vi "GDFgetEventTable.vi"(8 "error in (no error)":errorcluster, 11 "GDFv1.x in":refnum<class "GDFv1.x.lvclass">) -> (0 "error out":errorcluster, 2 "Event Table":T1[](array[typedef]), 3 "GDFv1.x out":refnum<class "GDFv1.x.lvclass">)   [LabVIEW 2016, in "GDF File Reader.lvlib" / "GDFv1.x.lvclass"]
uses:
  GDFv1.x.lvclass
  EventDataType.ctl
  GDFv1.x.lvclass/GDFv1.x.ctl
  GDF File Reader.lvlib
panel:
  # "This VI is a part of BCI Design library, http://www.ru-bci.org \nCopyright © 2020, Sotnikov Peter, All rights reserved. License: GNU GPLv3"
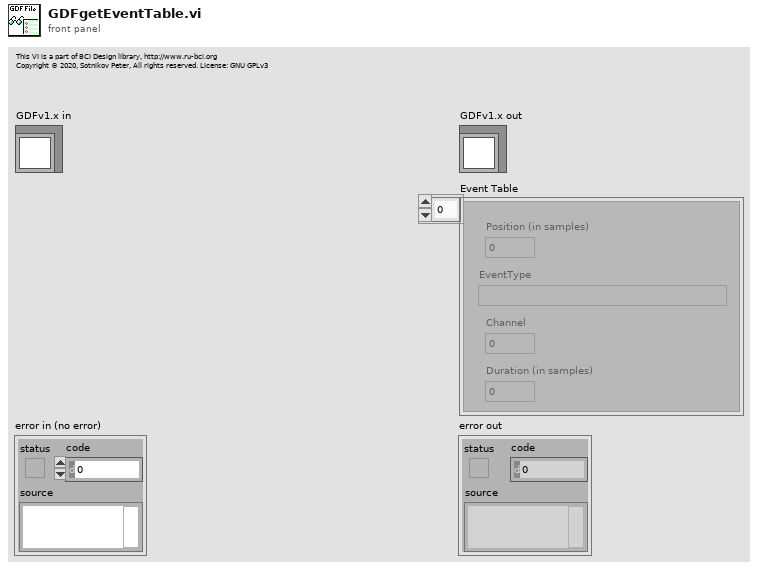
[diagram p1: front panel]
types:
  T1 = typedef "GDF File Reader.lvlib/EventDataType.ctl" = cluster{"Position (in samples)":u32, "EventType":string, "Channel":u16, "Duration (in samples)":u32}
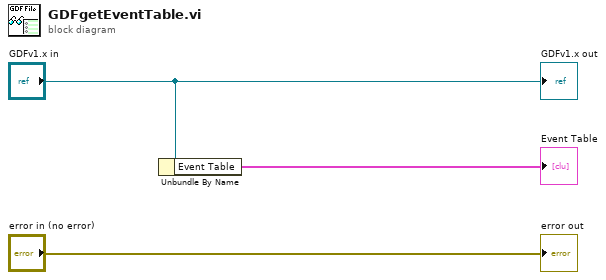
[diagram p0: block diagram]
diagram:
  n1 = Unbundle By Name("GDFv1.x in") -> ("Event Table"=→"Event Table":T1[])
  "error out" <- "error in (no error)"
  "GDFv1.x out" <- "GDFv1.x in"
